vi "Utility - Generate IO Variable Arrays.vi"() -> ()   [LabVIEW 2018, in "Outputs.lvlib"]
uses:
  Outputs.lvlib
panel:
  out "02-05":refnum<k21>[](array[refnum])
  out "02-01":refnum<k21>[](array[refnum])
  out "02-00":refnum<k21>[](array[refnum])
  out "02-06":refnum<k21>[](array[refnum])
  out "02-03":refnum<k21>[](array[refnum])
  out "02-02":refnum<k21>[](array[refnum])
  out "01-02":refnum<k21>[](array[refnum])
  out "01-01":refnum<k21>[](array[refnum])
  out "01-00":refnum<k21>[](array[refnum])
  out "00-01":refnum<k21>[](array[refnum])
  out "00-00":refnum<k21>[](array[refnum])
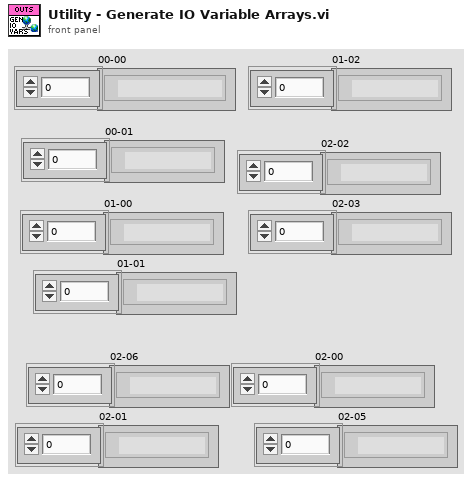
[diagram p1: front panel]
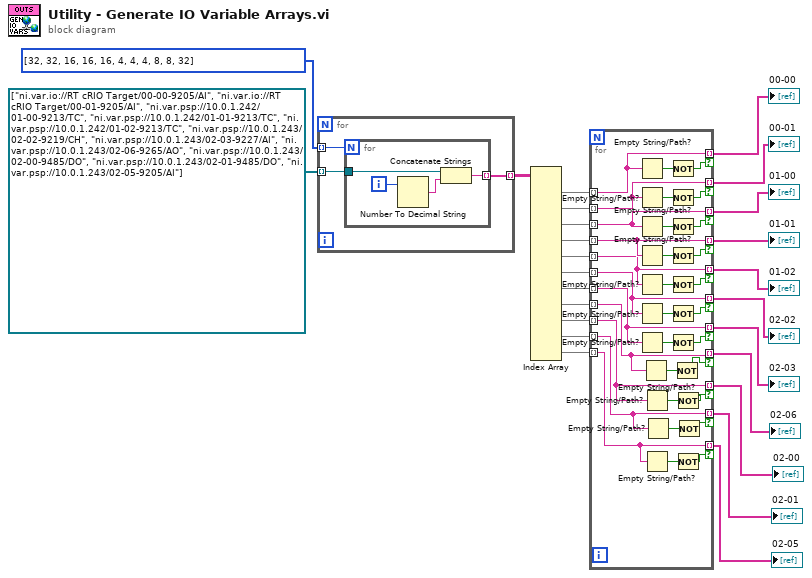
[diagram p0: block diagram]
diagram:
  n1 = for {
    tunnel: refnum<k21>[] ["ni.var.io://RT cRIO Target/00-00-9205/AI", "ni.var.io://RT cRIO Target/00-01-9205/AI", "ni.var.psp://10.0.1.242/01-00-9213/TC", "ni.var.psp://10.0.1.242/01-01-9213/TC", "ni.var.psp://10.0.1.242/01-02-9213/TC", "ni.var.psp://10.0.1.243/02-02-9219/CH", "ni.var.psp://10.0.1.243/02-03-9227/AI", "ni.var.psp://10.0.1.243/02-06-9265/AO", "ni.var.psp://10.0.1.243/02-00-9485/DO", "ni.var.psp://10.0.1.243/02-01-9485/DO", "ni.var.psp://10.0.1.243/02-05-9205/AI"] -> [w28] mode=indexing
    tunnel: i32[] [32, 32, 16, 16, 16, 4, 4, 4, 8, 8, 32] -> [w27] mode=indexing
    tunnel: [w26] -> w25 mode=indexing
    n2 = for {
      N: w27 -> [_]
      tunnel: w28 -> [w31]
      tunnel: [w29] -> w26 mode=indexing
      i -> [w32]
      n3 = Number To Decimal String(number=w32) -> (decimal integer string=w30:string)  [unwired: 1 in]
      n4 = Concatenate Strings(w31, w30) -> (w29:string)
    }
  }
  n5 = Index Array(array=w25) -> (element #1=w18:string[], element #2=w19:string[], element #3=w20:string[], element #4=w21:string[], element #5=w22:string[], element #6=w23:string[], element #7=w24:string[], element #8=w8:string[], element #9=w7:string[], element #10=w6:string[], element #11=w2:string[])  [unwired: 22 in]
  n6 = for {
    tunnel: w18 -> [w65] mode=indexing
    tunnel: [w65] -> w15 mode=indexing if=w51
    tunnel: w19 -> [w63] mode=indexing
    tunnel: w20 -> [w62] mode=indexing
    tunnel: w21 -> [w61] mode=indexing
    tunnel: w22 -> [w60] mode=indexing
    tunnel: w23 -> [w59] mode=indexing
    tunnel: w24 -> [w58] mode=indexing
    tunnel: [w63] -> w14 mode=indexing if=w50
    tunnel: [w62] -> w13 mode=indexing if=w49
    tunnel: [w61] -> w12 mode=indexing if=w48
    tunnel: [w60] -> w11 mode=indexing if=w47
    tunnel: [w59] -> w10 mode=indexing if=w46
    tunnel: [w58] -> w9 mode=indexing if=w45
    tunnel: w8 -> [w40] mode=indexing
    tunnel: w7 -> [w41] mode=indexing
    tunnel: [w40] -> w5 mode=indexing if=w36
    tunnel: [w41] -> w4 mode=indexing if=w37
    tunnel: w6 -> [w39] mode=indexing
    tunnel: [w39] -> w3 mode=indexing if=w38
    tunnel: w2 -> [w33] mode=indexing
    tunnel: [w33] -> w1 mode=indexing if=w34
    n7 = Empty String/Path?(string/path=w65) -> (empty?=w64:bool)
    n8 = Empty String/Path?(string/path=w63) -> (empty?=w57:bool)
    n9 = Empty String/Path?(string/path=w62) -> (empty?=w56:bool)
    n10 = Empty String/Path?(string/path=w61) -> (empty?=w55:bool)
    n11 = Empty String/Path?(string/path=w60) -> (empty?=w54:bool)
    n12 = Empty String/Path?(string/path=w59) -> (empty?=w53:bool)
    n13 = Empty String/Path?(string/path=w58) -> (empty?=w52:bool)
    n14 = Empty String/Path?(string/path=w40) -> (empty?=w44:bool)
    n15 = Empty String/Path?(string/path=w41) -> (empty?=w43:bool)
    n16 = Empty String/Path?(string/path=w33) -> (empty?=w35:bool)
    n17 = Empty String/Path?(string/path=w39) -> (empty?=w42:bool)
    n18 = Not(x=w64) -> (.not. x?=w51:bool)
    n19 = Not(x=w57) -> (.not. x?=w50:bool)
    n20 = Not(x=w56) -> (.not. x?=w49:bool)
    n21 = Not(x=w55) -> (.not. x?=w48:bool)
    n22 = Not(x=w54) -> (.not. x?=w47:bool)
    n23 = Not(x=w53) -> (.not. x?=w46:bool)
    n24 = Not(x=w52) -> (.not. x?=w45:bool)
    n25 = Not(x=w44) -> (.not. x?=w36:bool)
    n26 = Not(x=w43) -> (.not. x?=w37:bool)
    n27 = Not(x=w35) -> (.not. x?=w34:bool)
    n28 = Not(x=w42) -> (.not. x?=w38:bool)
  }
  "00-00" <- w15
  "00-01" <- w14
  "01-00" <- w13
  "01-01" <- w12
  "01-02" <- w11
  "02-02" <- w10
  "02-03" <- w9
  "02-06" <- w5
  "02-00" <- w4
  "02-01" <- w3
  "02-05" <- w1
